vi "Triggering DIO state.vi"(8 "error in (no error)":errorcluster, 9 "level":bool=TRUE, 10 "pin":T1 items=["DIO1"=1, "DIO2"=2, "DIO3"=3, "DIO4"=4, "DIO5"=5, "DIO6"=6, "DIO7"=7, "DIO8"=8], 11 "MicroDAQ.lvlib:Analog Input.lvclass":refnum<class "Analog Input.lvclass">) -> (0 "error out":errorcluster, 3 "MicroDAQ.lvlib:Analog Input.lvclass out":refnum<class "Analog Input.lvclass">)   [LabVIEW 2009, in "MicroDAQ.lvlib" / "Analog Input.lvclass"]
doc: "With this trigger task will start when given level (state) will occure on given digital input (pin)."
uses:
  <instrlib>/MicroDAQ/Channel/Analog Input/Analog Input.lvclass
  <instrlib>/MicroDAQ/Tools/Trigger DIO ring.ctl
  <instrlib>/MicroDAQ/Tools/Trigger type.ctl
  <instrlib>/MicroDAQ/Mlink library wraper/mlink.lvlib
  <instrlib>/MicroDAQ/Channel/Channel.lvclass
  <instrlib>/MicroDAQ/MicroDAQ.lvlib
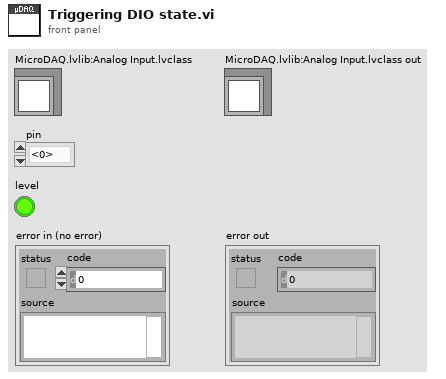
[diagram p1: front panel]
types:
  T1 = typedef "MicroDAQ.lvlib/Trigger DIO ring.ctl" = u16
  T2 = typedef "MicroDAQ.lvlib/Trigger type.ctl" = enum8{"Analog output", "Analog input"}
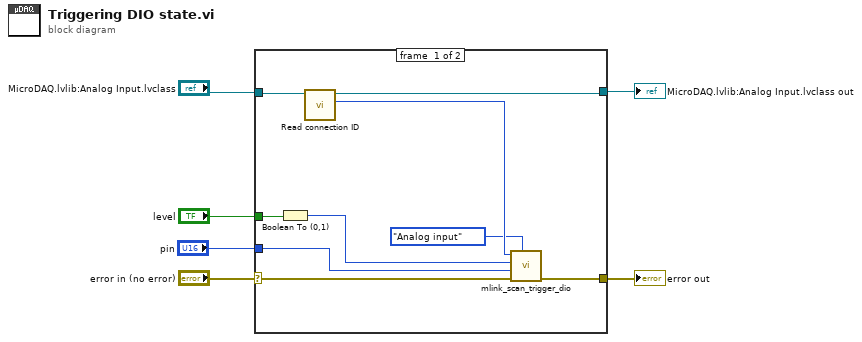
[diagram p0: block diagram]
diagram:
  n1 = case shown="No Error" "error in (no error)" {
    selector: "error in (no error)" -> [w13 w16]
    tunnel: [w12 w16] -> w5
    tunnel: [w14 w17] -> w4
    tunnel: "MicroDAQ.lvlib:Analog Input.lvclass" -> [w15 w17]
    tunnel: "pin" -> [w9 _]
    tunnel: "level" -> [w8 _]
    frame #0 {
      n2 = Boolean To (0,1)(Boolean=w8) -> (0, 1=w7:i16)
      n3 = call <instrlib>:"Read connection ID.vi"("Task in"=w15) -> ("connection ID"=w11:i32, "Task out"=w14:refnum<class "Analog Input.lvclass">)  [unwired: 9 in]
      n4 = call <instrlib>:"mlink_scan_trigger_dio.vi"("trigger type"=Trigger_type."Analog input", "error in (no error)"=w13, "dio"=w9, "level"=w7, "connection ID"=w11) -> ("error out"=w12:errorcluster)  [unwired: 5 in, 1 out]
    }
    frame #1 {
    }
  }
  "error out" <- w5
  "MicroDAQ.lvlib:Analog Input.lvclass out" <- w4
